vi "Queuedriver_producerconsumer.vi"(8 "error in":errorcluster, 9 "Operation":T2, 11 "Array":T1[](array[typedef])) -> (0 "error in 2":errorcluster, 3 "Enum":T1=enum."Start task")   [LabVIEW 2011]
uses:
  Control 2.ctl
  Control.ctl
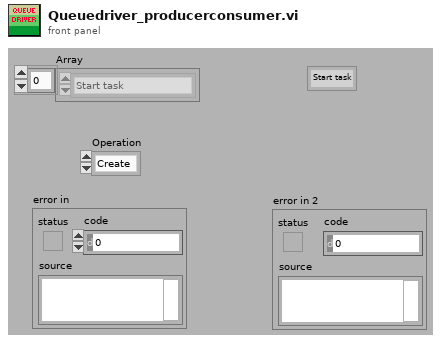
[diagram p1: front panel]
types:
  T1 = typedef "Control 2.ctl" = enum16{"Initialize", "Initialize_2", "Poll", "Start task", "Change states", "Exit"}
  T2 = typedef "Control.ctl" = enum16{"Create", "Enqueue-N", "Dequeue - 1 ", "Enstack - N", "Flush", "Release"}
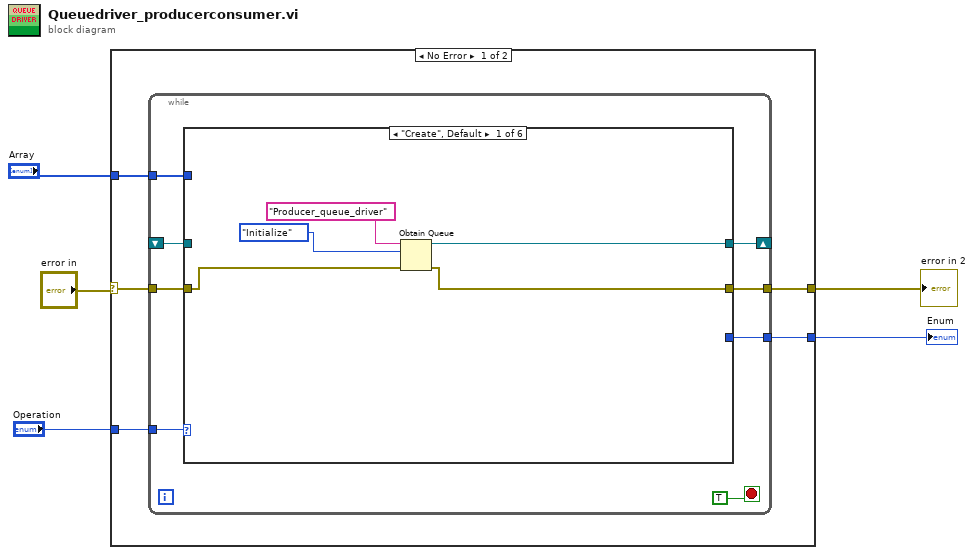
[diagram p0: block diagram]
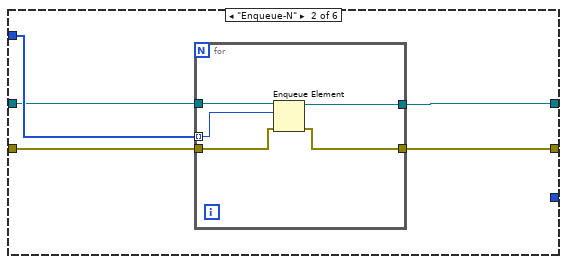
[diagram p2: hidden frame]
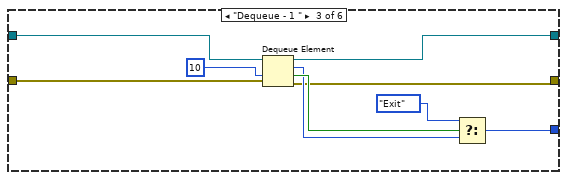
[diagram p3: hidden frame]
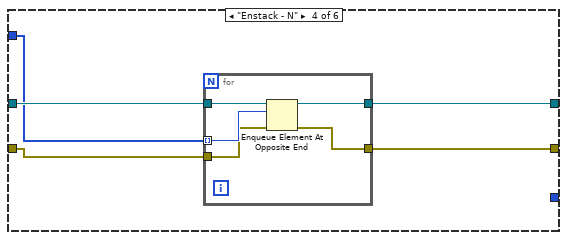
[diagram p4: hidden frame]
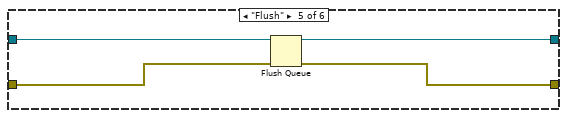
[diagram p5: hidden frame]
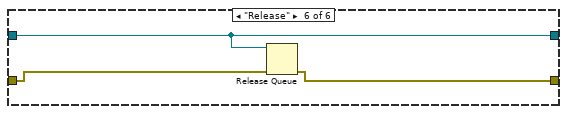
[diagram p6: hidden frame]
diagram:
  n1 = case shown="No Error" "error in" {
    selector: "error in" -> [w8 w60]
    tunnel: "Array" -> [w10 _]
    tunnel: "Operation" -> [w9 _]
    tunnel: [w7 w60] -> w2
    tunnel: [w6 _] -> w1
    frame No Error {
      n2 = while {
        tunnel: w10 -> [w17]
        tunnel: w9 -> [w16]
        tunnel: w8 -> [w15]
        tunnel: [w14] -> w7
        shift-right: [w13] -> _
        shift-left: _ -> [w12]
        tunnel: [w11] -> w6
        stop <- TRUE stop-if-true
        n3 = case shown="\"Create\", Default" w16 {
          tunnel: w17 -> [_ w28 _ w45 _ _]
          tunnel: w15 -> [w22 w27 w42 w44 w54 w58]
          tunnel: [w20 w26 w35 w43 w53 w57] -> w14
          tunnel: [w21 w25 w37 w46 w55 w59] -> w13
          tunnel: w12 -> [_ w24 w38 w47 w56 w59]
          tunnel: [_ _ w36 _ _ _] -> w11
          frame "Create", Default {
            n4 = Obtain Queue(name (unnamed)="Producer_queue_driver", element data type=Control_2."Initialize" ("Enum 2"), error in (no error)=w22) -> (queue out=w21:refnum<queue>, error out=w20:errorcluster)  [unwired: 2 in, 1 out]
          }
          frame "Enqueue-N" {
            n5 = for {
              tunnel: w28 -> [w32] mode=indexing
              tunnel: w24 -> [w33]
              tunnel: w27 -> [w30]
              tunnel: [w29] -> w26
              tunnel: [w31] -> w25
              n6 = Enqueue Element(queue=w33, element=w32, error in (no error)=w30) -> (queue out=w31:refnum<queue>, error out=w29:errorcluster)  [unwired: 1 in, 1 out]
            }
          }
          frame "Dequeue - 1 " {
            n7 = Dequeue Element(queue=w38, timeout in ms (-1)=10, error in (no error)=w42) -> (queue out=w37:refnum<queue>, element=w39:T1, timed out?=w40:bool, error out=w35:errorcluster)
            n8 = Select(t=Control_2."Exit" ("Enum 2"), s=w40, f=w39) -> (s? t:f=w36:T1)
          }
          frame "Enstack - N" {
            n9 = for {
              tunnel: w47 -> [w52]
              tunnel: [w51] -> w46
              tunnel: w45 -> [w50] mode=indexing
              tunnel: w44 -> [w49]
              tunnel: [w48] -> w43
              n10 = Enqueue Element At Opposite End(queue=w52, element=w50, error in (no error)=w49) -> (queue out=w51:refnum<queue>, error out=w48:errorcluster)  [unwired: 1 in, 1 out]
            }
          }
          frame "Flush" {
            n11 = Flush Queue(queue=w56, error in (no error)=w54) -> (queue out=w55:refnum<queue>, error out=w53:errorcluster)  [unwired: 1 out]
          }
          frame "Release" {
            n12 = Release Queue(queue=w59, error in (no error)=w58) -> (error out=w57:errorcluster)  [unwired: 1 in, 2 out]
          }
        }
      }
    }
    frame Error {
    }
  }
  "error in 2" <- w2
  "Enum" <- w1
